vi "pcfs_DO_perform_scan.vi"(8 "error in (no error)":errorcluster, 10 "scan_position_settings":T1={"Center Pos. (mm)"=0.0, "Increment (mm)"=0.0, "Steps"=0.0, "Dither Dist (nm)"=0.0, "Dither Period (s)"=0.0, "Cycles"=0.0, "Record Type"=enum."hdf5", "Save Path"=path "", "Stage Number"=enum."1", "File Notes"="", "Mode"=2, "overwrite"=FALSE, "custom_path"=FALSE, "custom_positions"=[]} {"Mode" items=["T2"=2, "T3"=3]}, 11 "scan_panel in":refnum<class "pcfs.lvclass">) -> (0 "error out":errorcluster, 3 "scan_panel out":refnum<class "pcfs.lvclass">)   [LabVIEW 2015, in "pcfs.lvclass"]
uses:
  pcfs.lvclass
  pcfs_settings.ctl
  Scan/scan_record.ctl
  Detector_Class/Picoquant/Hydraharp/hydraharp_panel/hpanel_acq_modes.ctl
  pcfs_position_settings.ctl
  Stage Class/Newport XPS/newport_xps/dither_trajectory_settings.ctl
  Stage Class/Newport XPS/newport_xps/dither_trajectory_types.ctl
  UI/front_panel_class/hardware_caller_queue_numbers.ctl
  Stage Class/Stage.lvclass
  Detector_Class/detector/detector.lvclass
  pcfs_log/pcfs_hdf5_log.lvclass
  spcfs_fsm_tasks.ctl
  pcfs.lvclass/pcfs.ctl
  Data Logger Class/data_logger.lvclass
  UI/panel_class/panel.lvclass
panel:
  out "error out 3":errorcluster
  out "error out 2":errorcluster
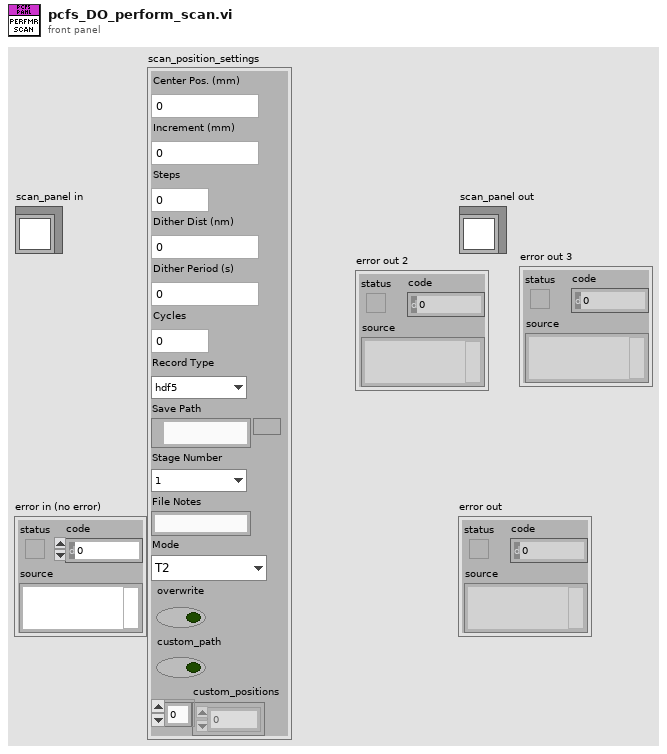
[diagram p1: front panel]
types:
  T1 = typedef "pcfs_settings.ctl" = cluster{"Center Pos. (mm)":dbl, "Increment (mm)":dbl, "Steps":dbl, "Dither Dist (nm)":dbl, "Dither Period (s)":dbl, "Cycles":dbl, "Record Type":T2, "Save Path":path, "Stage Number":enum16{"1", "2"}, "File Notes":string, "Mode":T3, "overwrite":bool, "custom_path":bool, "custom_positions":dbl[]}
  T2 = typedef "scan_record.ctl" = enum16{"hdf5", "legacy", "None"}
  T3 = typedef "hpanel_acq_modes.ctl" = u16
  T4 = typedef "dither_trajectory_types.ctl" = enum16{"Sawtooth"}
  T5 = typedef "dither_trajectory_settings.ctl" = cluster{"PVT Ampl (nm)":dbl, "Dither Period (s)":dbl, "Type":T4, "Name":string}
  T6 = typedef "pcfs_position_settings.ctl" = cluster{"Center Pos. (mm)":dbl, "increment":dbl, "steps":dbl, "dither_dist":dbl, "dither_period":dbl}
  T7 = typedef "spcfs_fsm_tasks.ctl" = enum16{"move stage, start dither", "collect stream", "stop dither", "finish_position"}
  T8 = typedef "hardware_caller_queue_numbers.ctl" = enum16{"stage1", "stage2", "experiment", "detector"}
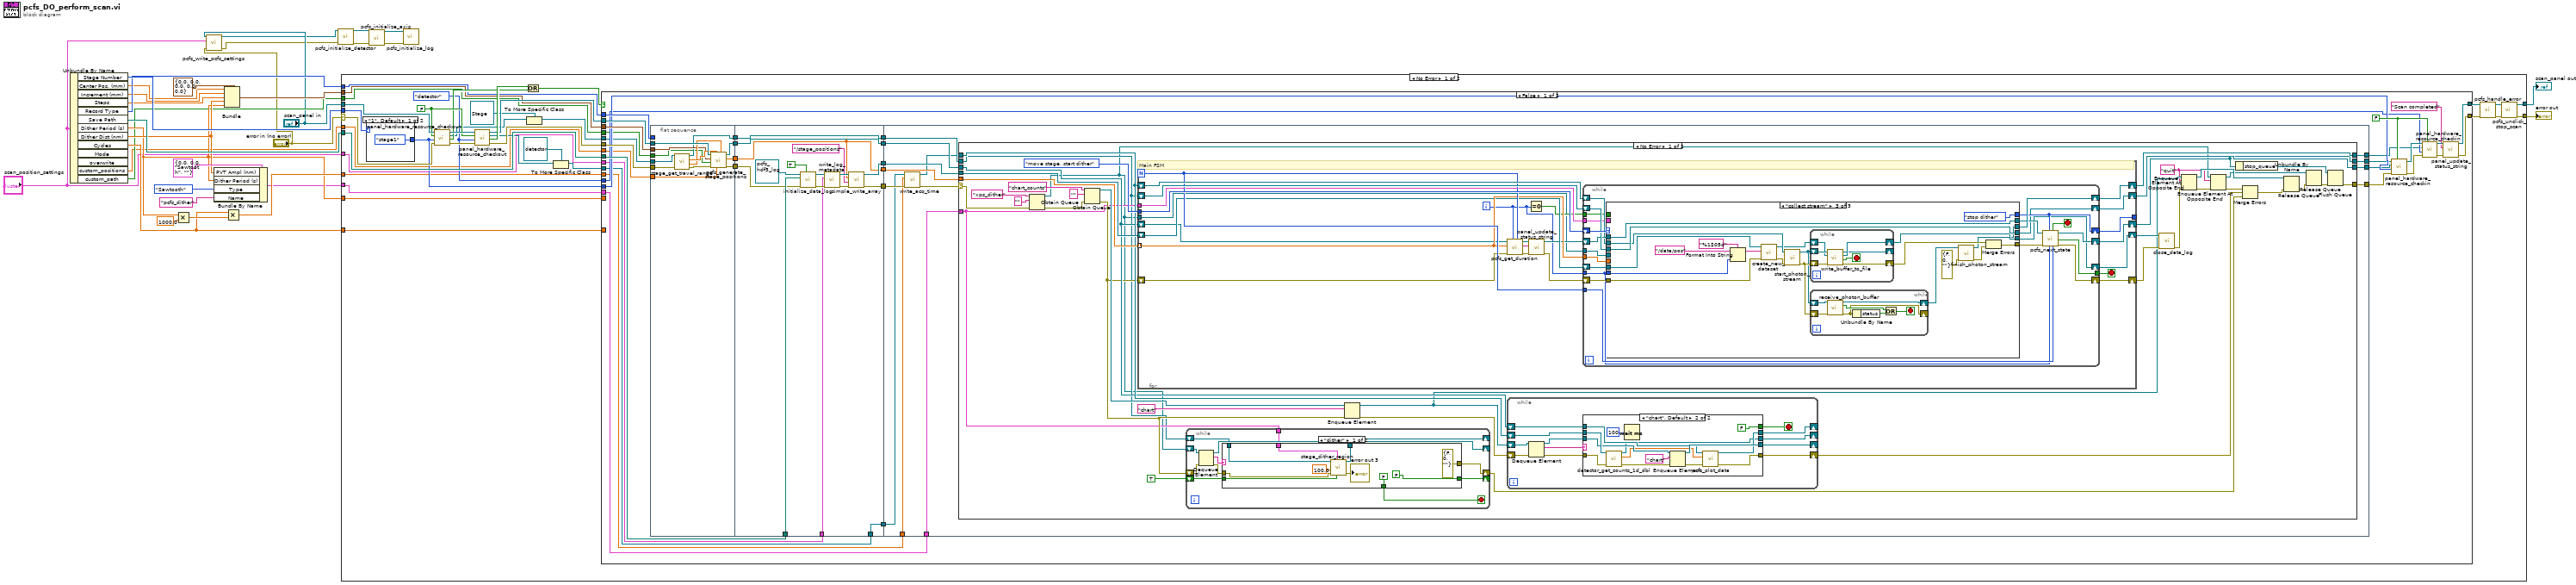
[diagram p0: block diagram]
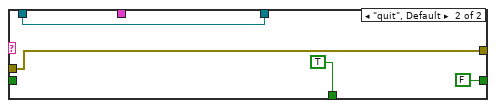
[diagram p2: hidden frame]
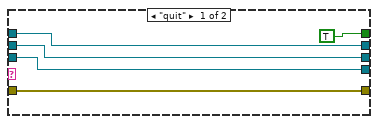
[diagram p3: hidden frame]
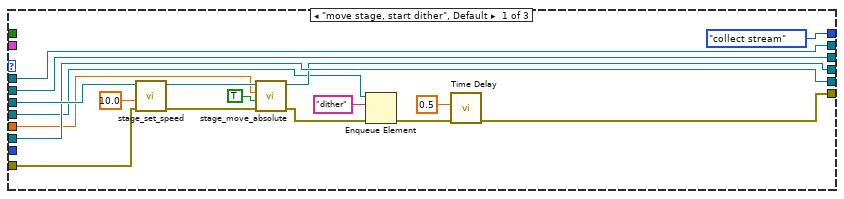
[diagram p4: hidden frame]
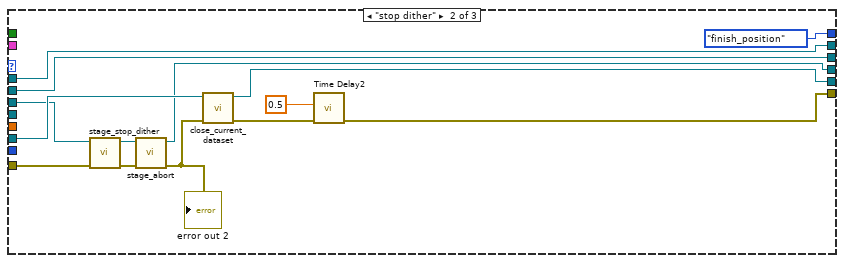
[diagram p5: hidden frame]
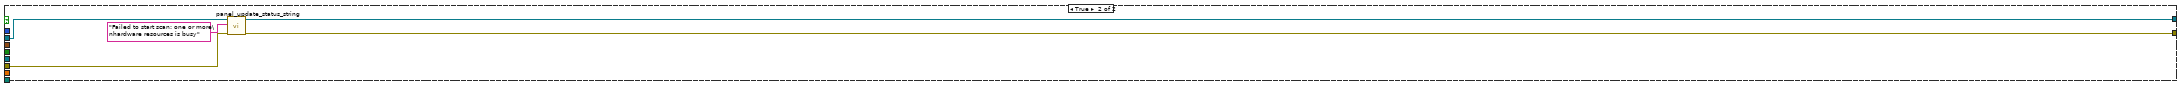
[diagram p7: hidden frame]
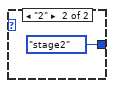
[diagram p8: hidden frame]
diagram:
  n1 = Unbundle By Name("scan_position_settings") -> ("Stage Number"=w29:enum16{"1", "2"}, "Center Pos. (mm)"=w24:dbl, "Increment (mm)"=w23:dbl, "Steps"=w22:dbl, "Record Type"=w27:T2, "Save Path"=w26:path, "Dither Period (s)"=w15:dbl, "Dither Dist (nm)"=w16:dbl, "Cycles"=w18:dbl, "custom_positions"=w10:dbl[], "custom_path"=w11:bool)  [unwired: 2 out]
  n2 = Multiply(x=w15, y=1000.0) -> (x*y=w20:dbl)
  n3 = call "pcfs_write_pcfs_settings.vi"("error in (no error)"="error in (no error)", "pcfs_settings"="scan_position_settings", "pcfs in"="scan_panel in") -> ("error out"=w6:errorcluster, "pcfs out"=w5:refnum<class "pcfs.lvclass">)  [unwired: 7 in]
  n4 = Bundle By Name(cluster=T5 {"PVT Ampl (nm)"=0.0, "Dither Period (s)"=0.0, "Type"=enum."Sawtooth", "Name"=""} ("Custom Dither Trajectory"), "PVT Ampl (nm)"=w16, "Dither Period (s)"=w15, "Type"=dither_trajectory_types."Sawtooth", "Name"="pcfs_dither") -> (w12:T5)
  n5 = Bundle(cluster=T6 {"Center Pos. (mm)"=0.0, "increment"=0.0, "steps"=0.0, "dither_dist"=0.0, "dither_period"=0.0} ("scan_position_settings"), "Center Pos. (mm)"=w24, "increment"=w23, "steps"=w22, "dither_dist"=w16, "dither_period"=w15) -> (w28:T6)
  n6 = Multiply(x=w18, y=w20) -> (x*y=w19:dbl)
  n7 = call "pcfs_initialize_detector.vi"("error in (no error)"=w6, "pcfs in"=w5) -> ("error out"=w4:errorcluster, "pcfs out"=w3:refnum<class "pcfs.lvclass">)  [unwired: 8 in]
  n8 = case shown="No Error" "error in (no error)" {
    selector: "error in (no error)" -> [w66 w366]
    tunnel: [w40 w366] -> w31
    tunnel: [w41 w365] -> w30
    tunnel: "scan_panel in" -> [w64 w365]
    tunnel: w29 -> [w65 _]
    tunnel: w28 -> [w55 _]
    tunnel: w27 -> [w54 _]
    tunnel: w26 -> [w53 _]
    tunnel: "scan_position_settings" -> [w38 _]
    tunnel: w19 -> [w37 _]
    tunnel: w15 -> [w36 _]
    tunnel: w18 -> [w35 _]
    tunnel: w12 -> [w34 _]
    tunnel: w11 -> [w33 _]
    tunnel: w10 -> [w32 _]
    frame No Error {
      w45 = hardware_caller_queue_numbers."detector" ("panel_number")
      w61 = FALSE ("Self?")
      n9 = case shown="\"1\", Default" w65 {
        tunnel: [hardware_caller_queue_numbers."stage1" ("panel_number") hardware_caller_queue_numbers."stage2" ("panel_number")] -> w46
        frame "1", Default {
        }
        frame "2" {
        }
      }
      n10 = call "panel_hardware_resource_checkout.vi"("error in (no error)"=w66, "panel_number"=w46, "Self?"=w61, "panel in"=w64) -> ("error out"=w63:errorcluster, "timed out?"=w59:bool, "hardware.lvclass"=w52:refnum<class "hardware.lvclass">, "panel out"=w62:refnum<class "pcfs.lvclass">)  [unwired: 4 in]
      n11 = call "panel_hardware_resource_checkout.vi"("error in (no error)"=w63, "panel_number"=w45, "Self?"=w61, "panel in"=w62) -> ("error out"=w57:errorcluster, "timed out?"=w60:bool, "hardware.lvclass"=w49:refnum<class "hardware.lvclass">, "panel out"=w56:refnum<class "pcfs.lvclass">)  [unwired: 4 in]
      n12 = Or(x=w60, y=w59) -> (x .or. y?=w58:bool)
      n13 = To More Specific Class(target class=refnum<class "Stage.lvclass"> refnum ("Stage.lvclass"), reference=w52) -> (specific class reference=w50:refnum<class "Stage.lvclass">)  [unwired: 1 in, 1 out]
      n14 = To More Specific Class(target class=refnum<class "detector.lvclass"> refnum ("detector.lvclass"), reference=w49) -> (specific class reference=w47:refnum<class "detector.lvclass">)  [unwired: 1 in, 1 out]
      n15 = case shown="False" w58 {
        tunnel: w57 -> [w99 w362]
        tunnel: w56 -> [w98 w360]
        tunnel: [w87 w359] -> w39
        tunnel: [w89 w361] -> w44
        tunnel: w55 -> [w97 _]
        tunnel: w54 -> [w96 _]
        tunnel: w53 -> [w95 _]
        tunnel: w50 -> [w85 _]
        tunnel: w47 -> [w80 _]
        tunnel: w46 -> [w92 _]
        tunnel: w45 -> [w91 _]
        tunnel: w38 -> [w71 _]
        tunnel: w37 -> [w70 _]
        tunnel: w36 -> [_ _]
        tunnel: w35 -> [_ _]
        tunnel: w34 -> [w69 _]
        tunnel: w33 -> [w68 _]
        tunnel: w32 -> [w67 _]
        frame False {
          w100 = FALSE ("Self")
          n16 = flat-sequence {
            tunnel: w99 -> [w113]
            tunnel: w98 -> [w115]
            tunnel: w97 -> [w108]
            tunnel: w96 -> [_]
            tunnel: [w114] -> w94
            tunnel: w85 -> [w111]
            tunnel: [w107] -> w83
            tunnel: [w106] -> w81
            tunnel: [w105] -> w78
            tunnel: w68 -> [w104]
            tunnel: w67 -> [w103]
            tunnel: w95 -> [w128]
            tunnel: w94 -> [w119]
            tunnel: w80 -> [w117]
            tunnel: [w119] -> w93
            tunnel: [w123] -> w84
            tunnel: w83 -> [w116]
            tunnel: [w131] -> w82
            tunnel: w81 -> [w131]
            tunnel: [w130] -> w79
            tunnel: w78 -> [w130]
            tunnel: [w117] -> w77
            tunnel: [w122] -> w72
            tunnel: w71 -> [w124]
            tunnel: w93 -> [w145]
            tunnel: w84 -> [w137]
            tunnel: w82 -> [w143]
            tunnel: w79 -> [w144]
            tunnel: w77 -> [w135]
            tunnel: [w142] -> w76
            tunnel: [w141] -> w75
            tunnel: [w140] -> w74
            tunnel: [w139] -> w73
            tunnel: w72 -> [w138]
            tunnel: w70 -> [w133]
            tunnel: w69 -> [w132]
            frame #0 {
              n17 = call-dynamic "stage_get_travel_range.vi"("error in (no error)"=w113, "Stage in"=w111) -> ("error out"=w112:errorcluster, "min(mm)"=w109:dbl, "max (mm)"=w110:dbl, "Stage out"=w105:refnum<class "Stage.lvclass">)  [unwired: 6 in]
              n18 = call "pcfs_generate_stage_positions.vi"("travel_min (mm)"=w109, "custom_positions"=w103, "travel_max (mm)"=w110, "error in (no error)"=w112, "custom_trajectory"=w104, "pcfs_settings"=w108, "scan_panel in"=w115) -> ("error out"=w107:errorcluster, "Positions (mm)"=w114:dbl[], "scan_panel out"=w106:refnum<class "pcfs.lvclass">)  [unwired: 2 out]
            }
            frame #1 {
              n19 = call-dynamic "initialize_data_log.vi"("Overwrite?"=TRUE, "error in (no error)"=w116, "Path"=w128, "pcfs_hdf5_log in"=refnum<class "pcfs_hdf5_log.lvclass"> refnum) -> ("error out"=w126:errorcluster, "pcfs_hdf5_log out"=w125:refnum<class "pcfs_hdf5_log.lvclass">)  [unwired: 6 in]
              n20 = call-dynamic "write_log_metadata.vi"("error in (no error)"=w126, "data"=w124, "pcfs_hdf5_log in"=w125) -> ("error out"=w120:errorcluster, "pcfs_hdf5_log out"=w121:refnum<class "pcfs_hdf5_log.lvclass">)  [unwired: 7 in]
              n21 = call-dynamic "simple_write_array.vi"("error in (no error)"=w120, "path"="/stage_positions", "Array"=w119, "pcfs_hdf5_log in"=w121) -> ("error out"=w123:errorcluster, "pcfs_hdf5_log out"=w122:refnum<class "pcfs_hdf5_log.lvclass">)  [unwired: 6 in]
            }
            frame #2 {
              n22 = call-dynamic "write_acq_time.vi"("error in (no error)"=w137, "acq_time"=w133, "detector in"=w135) -> ("error out"=w136:errorcluster, "detector out"=w134:refnum<class "detector.lvclass">)  [unwired: 7 in]
              n23 = case shown="No Error" w136 {
                selector: w136 -> [w161 w354]
                tunnel: w145 -> [w182 _]
                tunnel: w144 -> [w147 w356]
                tunnel: w143 -> [w170 w357]
                tunnel: w134 -> [w171 w355]
                tunnel: [w174 w354] -> w142
                tunnel: [w181 w355] -> w141
                tunnel: [w180 w356] -> w140
                tunnel: [w176 w357] -> w139
                tunnel: w138 -> [w179 _]
                tunnel: w132 -> [w148 _]
                frame No Error {
                  w154 = "quit" ("element")
                  n24 = Obtain Queue(name (unnamed)="xps_dither", element data type="", error in (no error)=w161) -> (queue out=w146:refnum<queue>, error out=w160:errorcluster)  [unwired: 2 in, 1 out]
                  n25 = Obtain Queue(name (unnamed)="chart_counts", element data type="", error in (no error)=w160) -> (queue out=w168:refnum<queue>, error out=w157:errorcluster)  [unwired: 2 in, 1 out]
                  n26 = for {
                    N -> [w255]
                    tunnel: w182 -> [w254] mode=indexing
                    shift-right: [w249] -> w178
                    shift-left: w157 -> [w250]
                    shift-right: [w251] -> w180
                    shift-left: w147 -> [w263]
                    shift-right: [w246] -> w176
                    shift-left: w170 -> [w248]
                    tunnel: spcfs_fsm_tasks."move stage, start dither" ("Enum") -> [w264]
                    tunnel: [w262] -> _
                    shift-right: [w260] -> w181
                    shift-left: w171 -> [w261]
                    shift-right: [w252] -> w177
                    shift-left: w179 -> [w253]
                    tunnel: w148 -> [w244]
                    tunnel: w146 -> [w241]
                    i -> [w243]
                    stop <- w259 stop-if-true
                    # "Main FSM"
                    n27 = call "pcfs_get_duration.vi"("total_steps"=w255, "current_iteration"=w243, "error in (no error)"=w250, "current_position"=w254, "scan_panel in"=w248) -> ("error out"=w258:errorcluster, "time_remaining"=w256:string, "scan_panel out"=w257:refnum<class "pcfs.lvclass">)  [unwired: 4 in]
                    n28 = Equal To 0?(x=w243) -> (x = 0?=w242:bool)
                    n29 = call-dynamic "panel_update_status_string.vi"("error in (no error)"=w258, "String"=w256, "scan_panel in"=w257) -> ("error out"=w245:errorcluster, "scan_panel out"=w247:refnum<class "pcfs.lvclass">)  [unwired: 7 in]
                    n30 = while {
                      tunnel: w254 -> [w285]
                      shift-right: [w274] -> w262
                      shift-left: w264 -> [w286]
                      shift-right: [w273] -> w246
                      shift-left: w247 -> [w282]
                      shift-right: [w269] -> w249
                      shift-left: w245 -> [w284]
                      shift-right: [w280] -> w260
                      shift-left: w261 -> [w281]
                      tunnel: w243 -> [w275]
                      tunnel: w255 -> [w279]
                      tunnel: [w272] -> w259
                      shift-right: [w270] -> w252
                      shift-left: w253 -> [w276]
                      shift-right: [w268] -> w251
                      shift-left: w263 -> [w283]
                      tunnel: w244 -> [w267]
                      tunnel: w242 -> [w266]
                      tunnel: w241 -> [w265]
                      stop <- w271 stop-if-true
                      n31 = case shown="\"collect stream\"" w286 {
                        tunnel: w285 -> [w292 _ _]
                        tunnel: w284 -> [w303 w313 w321]
                        tunnel: w283 -> [w302 w312 w338]
                        tunnel: [w297 w309 w319] -> w278
                        tunnel: w282 -> [w296 w317 w337]
                        tunnel: [w296 w317 w337] -> w277
                        tunnel: [spcfs_fsm_tasks."collect stream" ("Enum") spcfs_fsm_tasks."finish_position" ("Enum") spcfs_fsm_tasks."stop dither" ("Enum")] -> w274
                        tunnel: [w291 w305 w338] -> w268
                        tunnel: w281 -> [w294 w316 w333]
                        tunnel: [w294 w316 w327] -> w280
                        tunnel: w276 -> [w293 w315 w323]
                        tunnel: w275 -> [_ _ w335]
                        tunnel: [w293 w314 w329] -> w270
                        tunnel: w267 -> [_ _ _]
                        tunnel: w266 -> [_ _ _]
                        tunnel: w265 -> [w289 _ _]
                        frame "move stage, start dither", Default {
                          n32 = call-dynamic "stage_set_speed.vi"("error in (no error)"=w303, "Speed"=10.0, "Stage in"=w302) -> ("error out"=w301:errorcluster, "Stage out"=w300:refnum<class "Stage.lvclass">)  [unwired: 7 in]
                          n33 = call-dynamic "stage_move_absolute.vi"("error in (no error)"=w301, "wait_for_done"=TRUE, "Position"=w292, "Stage in"=w300) -> ("error out"=w290:errorcluster, "Stage out"=w291:refnum<class "Stage.lvclass">)  [unwired: 6 in]
                          n34 = Enqueue Element(queue=w289, element="dither", error in (no error)=w290) -> (error out=w287:errorcluster)  [unwired: 1 in, 2 out]
                          n35 = call "Time Delay"("error in (no error)"=w287, "Delay Time (s)"=0.5) -> ("error out"=w297:errorcluster)  [unwired: 9 in]
                        }
                        frame "stop dither" {
                          n36 = call-dynamic "stage_stop_dither.vi"("error in (no error)"=w313, "Stage in"=w312) -> ("error out"=w308:errorcluster, "Stage out"=w306:refnum<class "Stage.lvclass">)  [unwired: 8 in]
                          n37 = call-dynamic "stage_abort.vi"("error in (no error)"=w308, "Stage in"=w306) -> ("error out"=w307:errorcluster, "Stage out"=w305:refnum<class "Stage.lvclass">)  [unwired: 8 in]
                          "error out 2" <- w307
                          n38 = call-dynamic "close_current_dataset.vi"("error in (no error)"=w307, "data_logger in"=w315) -> ("error out"=w310:errorcluster, "data_logger out"=w314:refnum<class "data_logger.lvclass">)  [unwired: 8 in]
                          n39 = call "Time Delay2"("error in (no error)"=w310, "Delay Time (s)"=0.5) -> ("error out"=w309:errorcluster)  [unwired: 9 in]
                        }
                        frame "collect stream" {
                          n40 = Format Into String(format string="%1$05d", initial string="/data/pos" ("Path"), w335) -> (resulting string=w324:string)  [unwired: 1 in, 1 out]
                          n41 = call-dynamic "create_new_dataset.vi"("error in (no error)"=w321, "Path"=w324, "data_logger in"=w323) -> ("error out"=w325:errorcluster, "data_logger out"=w322:refnum<class "data_logger.lvclass">)  [unwired: 7 in]
                          n42 = call-dynamic "start_photon_stream.vi"("error in (no error)"=w325, "detector in"=w333) -> ("error out"=w332:errorcluster, "detector out"=w331:refnum<class "detector.lvclass">)  [unwired: 8 in]
                          n43 = while {
                            shift-right: [w341] -> w330
                            shift-left: w332 -> [w345]
                            shift-right: [w340] -> _
                            shift-left: w331 -> [w346]
                            shift-right: [w343] -> w329
                            shift-left: w322 -> [w344]
                            stop <- w342 stop-if-true
                            n44 = call-dynamic "write_buffer_to_file.vi"("error in (no error)"=w345, "data_logger.lvclass"=w344, "detector in"=w346) -> ("error out"=w341:errorcluster, "Stream_done"=w342:bool, "data_logger.lvclass 2"=w343:refnum<class "data_logger.lvclass">, "detector out"=w340:refnum<class "detector.lvclass">)  [unwired: 5 in]
                          }
                          n45 = while {
                            shift-right: [w348] -> _
                            shift-left: w332 -> [w347]
                            shift-right: [w349] -> w328
                            shift-left: w331 -> [w353]
                            stop <- w350 stop-if-true
                            n46 = call-dynamic "receive_photon_buffer.vi"("error in (no error)"=w347, "detector in"=w353) -> ("error out"=w348:errorcluster, "done"=w351:bool, "detector out"=w349:refnum<class "detector.lvclass">)  [unwired: 7 in]
                            n47 = Unbundle By Name(w348) -> ("status"=w352:bool)
                            n48 = Or(x=w351, y=w352) -> (x .or. y?=w350:bool)
                          }
                          n49 = call-dynamic "finish_photon_stream.vi"("error in (no error)"=errorcluster {"status"=FALSE, "code"=0, "source"=""}, "detector in"=w328) -> ("error out"=w326:errorcluster, "detector out"=w327:refnum<class "detector.lvclass">)  [unwired: 8 in]
                          n50 = Merge Errors(w330, w326) -> (w319:errorcluster)
                        }
                      }
                      n51 = call "pcfs_next_state.vi"("total_steps"=w279, "current_iteration"=w275, "next_state"=w274, "error in (no error)"=w278, "pcfs in"=w277) -> ("error out"=w269:errorcluster, "end_experiment"=w272:bool, "pcfs out"=w273:refnum<class "pcfs.lvclass">, "finish_position"=w271:bool)  [unwired: 3 in]
                    }
                  }
                  n52 = while {
                    shift-right: [w189] -> _
                    shift-left: w146 -> [w195]
                    shift-right: [w190] -> w153
                    shift-left: w157 -> [w194]
                    shift-right: [w187] -> _
                    shift-left: TRUE -> [w188]
                    tunnel: w148 -> [w186]
                    shift-right: [w184] -> _
                    shift-left: w147 -> [w185]
                    stop <- w192 stop-if-true
                    n53 = Dequeue Element(queue=w195, error in (no error)=w194) -> (queue out=w189:refnum<queue>, element=w193:string, error out=w191:errorcluster)  [unwired: 1 in, 1 out]
                    n54 = case shown="\"dither\"" w193 {
                      tunnel: [FALSE TRUE] -> w192
                      tunnel: w191 -> [w199 w208]
                      tunnel: [errorcluster {"status"=FALSE, "code"=0, "source"=""} ("error out") w208] -> w190
                      tunnel: w188 -> [w205 _]
                      tunnel: [FALSE FALSE] -> w187
                      tunnel: w186 -> [w203 _]
                      tunnel: w185 -> [w201 w206]
                      tunnel: [w200 w206] -> w184
                      frame "dither" {
                        n55 = call-dynamic "stage_dither_region.vi"("first_time?"=w205, "dither_params"=w203, "error in (no error)"=w199, "cycles"=100.0, "Stage in"=w201) -> ("error out"=→"error out 3":errorcluster, "Stage out"=w200:refnum<class "Stage.lvclass">)  [unwired: 5 in]
                      }
                      frame "quit", Default {
                      }
                    }
                  }
                  n56 = Enqueue Element(queue=w168, element="chart", error in (no error)=w157) -> (queue out=w164:refnum<queue>, error out=w169:errorcluster)  [unwired: 1 in, 1 out]
                  n57 = while {
                    shift-right: [w215] -> _
                    shift-left: w164 -> [w221]
                    shift-right: [w210] -> _
                    shift-left: w171 -> [w219]
                    shift-right: [w211] -> w166
                    shift-left: w169 -> [w220]
                    shift-right: [w212] -> _
                    shift-left: w170 -> [w213]
                    stop <- w214 stop-if-true
                    n58 = Dequeue Element(queue=w221, error in (no error)=w220) -> (queue out=w216:refnum<queue>, element=w218:string, error out=w217:errorcluster)  [unwired: 1 in, 1 out]
                    n59 = case shown="\"chart\", Default" w218 {
                      tunnel: w219 -> [w224 w240]
                      tunnel: w217 -> [w223 w239]
                      tunnel: w216 -> [w225 w237]
                      tunnel: [w225 w235] -> w215
                      tunnel: [TRUE FALSE] -> w214
                      tunnel: w213 -> [w222 w232]
                      tunnel: [w222 w230] -> w212
                      tunnel: [w223 w229] -> w211
                      tunnel: [w224 w228] -> w210
                      frame "quit" {
                      }
                      frame "chart", Default {
                        n60 = call-dynamic "detector_get_counts_1d_dbl.vi"("error in (no error)"=w239, "detector in"=w240) -> ("error out"=w238:errorcluster, "counts"=w231:dbl[], "detector out"=w228:refnum<class "detector.lvclass">)  [unwired: 7 in]
                        n61 = Wait (ms)(milliseconds to wait=u32 100) -> ()  [unwired: 1 out]
                        n62 = Enqueue Element(queue=w237, element="chart", error in (no error)=w238) -> (queue out=w235:refnum<queue>, error out=w233:errorcluster)  [unwired: 1 in, 1 out]
                        n63 = call "pcfs_plot_data.vi"("error in (no error)"=w233, "data"=w231, "scan_panel in"=w232) -> ("error out"=w229:errorcluster, "scan_panel out"=w230:refnum<class "pcfs.lvclass">)  [unwired: 7 in]
                      }
                    }
                  }
                  n64 = call-dynamic "close_data_log.vi"("error in (no error)"=w178, "data_logger in"=w177) -> ("error out"=w165:errorcluster)  [unwired: 8 in, 1 out]
                  n65 = Enqueue Element At Opposite End(queue=w164, element=w154, error in (no error)=w165) -> (queue out=w162:refnum<queue>, error out=w156:errorcluster)  [unwired: 1 in, 1 out]
                  n66 = Enqueue Element At Opposite End(queue=w146, element=w154, error in (no error)=w156) -> (queue out=w151:refnum<queue>, error out=w155:errorcluster)  [unwired: 1 in, 1 out]
                  n67 = Unbundle By Name(w176) -> ("stop_queue"=w175:refnum<queue>)
                  n68 = Merge Errors(w155, w166, w153) -> (w163:errorcluster)
                  n69 = Release Queue(queue=w162, error in (no error)=w163) -> (error out=w152:errorcluster)  [unwired: 1 in, 2 out]
                  n70 = Release Queue(queue=w151, error in (no error)=w152) -> (error out=w150:errorcluster)  [unwired: 1 in, 2 out]
                  n71 = Flush Queue(queue=w175, error in (no error)=w150) -> (error out=w174:errorcluster)  [unwired: 2 out]
                }
                frame Error {
                }
              }
            }
          }
          n72 = call "panel_hardware_resource_checkin.vi"("Self"=w100, "error in (no error)"=w76, "panel_number"=w92, "hardware.lvclass"=w74, "panel in"=w73) -> ("error out"=w102:errorcluster, "panel out"=w101:refnum<class "pcfs.lvclass">)  [unwired: 5 in]
          n73 = call "panel_hardware_resource_checkin.vi"("Self"=w100, "error in (no error)"=w102, "panel_number"=w91, "hardware.lvclass"=w75, "panel in"=w101) -> ("error out"=w90:errorcluster, "panel out"=w88:refnum<class "pcfs.lvclass">)  [unwired: 5 in]
          n74 = call-dynamic "panel_update_status_string.vi"("error in (no error)"=w90, "String"="Scan completed", "scan_panel in"=w88) -> ("error out"=w89:errorcluster, "scan_panel out"=w87:refnum<class "pcfs.lvclass">)  [unwired: 7 in]
        }
        frame True {
          n75 = call-dynamic "panel_update_status_string.vi"("error in (no error)"=w362, "String"="Failed to start scan: one or more\nhardware resources is busy", "scan_panel in"=w360) -> ("error out"=w361:errorcluster, "scan_panel out"=w359:refnum<class "pcfs.lvclass">)  [unwired: 7 in]
        }
      }
      n76 = call "pcfs_handle_error.vi"("error in (no error)"=w44, "scan_panel in"=w39) -> ("error out"=w43:errorcluster, "scan_panel out"=w42:refnum<class "pcfs.lvclass">)  [unwired: 8 in]
      n77 = call "pcfs_unclick_stop_scan.vi"("error in (no error)"=w43, "scan_panel in"=w42) -> ("error out"=w40:errorcluster, "scan_panel out"=w41:refnum<class "pcfs.lvclass">)  [unwired: 8 in]
    }
    frame Error {
    }
  }
  "error out" <- w31
  "scan_panel out" <- w30
  n78 = call "pcfs_initialize_axis.vi"("error in (no error)"=w4, "pcfs in"=w3) -> ("error out"=w2:errorcluster, "pcfs out"=w1:refnum<class "pcfs.lvclass">)  [unwired: 8 in]
  n79 = call "pcfs_initialize_log.vi"("error in (no error)"=w2, "pcfs in"=w1) -> ()  [unwired: 8 in, 2 out]
